vi "LJM_ListAllS.vi"(8 "error in":errorcluster, 10 "ConnectionType":string="LJM_ctUSB", 11 "DeviceType":string="LJM_dtT7") -> (0 "error out":errorcluster, 1 "aIPAddresses (IPv4Strings)":string[](array[string]), 2 "aIPAddresses":i32[](array[numeric]), 3 "aSerialNumbers":i32[](array[numeric]), 4 "aConnectionTypes":i32[](array[numeric]), 5 "NumFound":i32, 6 "aDeviceTypes":i32[](array[numeric]))   [LabVIEW 2020]
uses:
  LabJackM.framework
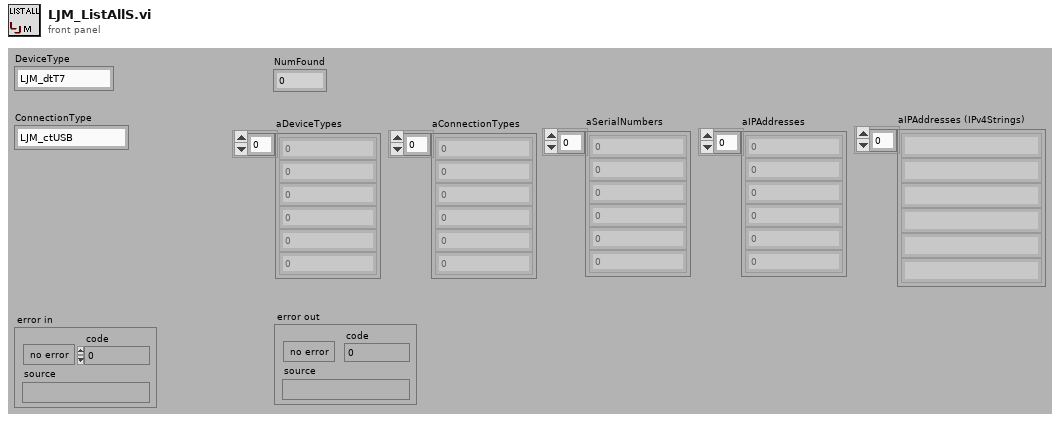
[diagram p1: front panel]
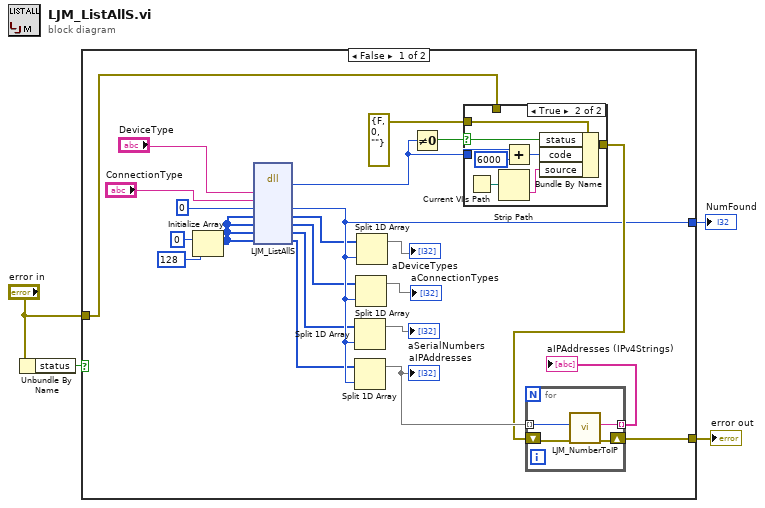
[diagram p0: block diagram]
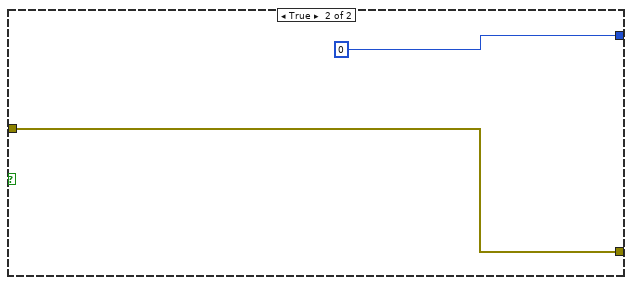
[diagram p3: hidden frame]
diagram:
  n1 = Unbundle By Name("error in") -> ("status"=w4:bool)
  n2 = case shown="False" w4 {
    tunnel: "error in" -> [w23 w41]
    tunnel: [w11 0 ("NumFound")] -> w2
    tunnel: [w13 w41] -> w1
    frame False {
      n3 = Initialize Array(0 ("element"), 128 ("dimension size")) -> (w12:i32[])
      n4 = dll-call lib="LabJackM.framework" fn="LJM_ListAllS"("DeviceType"="DeviceType", "ConnectionType"="ConnectionType", "NumFound"=0 ("Handle"), "aDeviceTypes"=w12, "aConnectionTypes"=w12, "aIPAddresses"=w12, "aSerialNumbers"=w12) -> ("return type"=w24:i32, "NumFound"=w11:i32, "aDeviceTypes"=w7:i32[], "aConnectionTypes"=w8:i32[], "aIPAddresses"=w9:i32[], "aSerialNumbers"=w10:i32[])  [unwired: 5 in, 2 out]
      n5 = Split 1D Array(array=w9, index=w11) -> (first subarray=→"aSerialNumbers":i32[])  [unwired: 1 out]
      n6 = Split 1D Array(array=w10, index=w11) -> (first subarray=w16:i32[])  [unwired: 1 out]
      "aIPAddresses" <- w16
      n7 = Split 1D Array(array=w8, index=w11) -> (first subarray=→"aConnectionTypes":i32[])  [unwired: 1 out]
      n8 = Split 1D Array(array=w7, index=w11) -> (first subarray=→"aDeviceTypes":i32[])  [unwired: 1 out]
      n9 = Not Equal To 0?(x=w24) -> (x != 0?=w25:bool)
      n10 = case shown="True" w25 {
        selector: w25 -> [_ w38]
        tunnel: [w31 w39] -> w14
        tunnel: errorcluster {"status"=FALSE, "code"=0, "source"=""} ("error IO") -> [_ w37]
        tunnel: w24 -> [_ w33]
        tunnel: w23 -> [w31 _]
        frame False {
        }
        frame True {
          n11 = Current VI's Path() -> (path=w35:path)
          n12 = Strip Path(path=w35) -> (name=w36:string)  [unwired: 1 out]
          n13 = Add(x=w33, y=6000) -> (x+y=w34:i32)
          n14 = Bundle By Name(cluster=w37, "status"=w38, "code"=w34, "source"=w36) -> (w39:errorcluster)
        }
      }
      n15 = for {
        tunnel: w16 -> [w30] mode=indexing
        tunnel: [w29] -> w15 mode=indexing
        shift-right: [w27] -> w13
        shift-left: w14 -> [w28]
        n16 = call "LJM_NumberToIP.vi"("error in"=w28, "Number"=w30) -> ("error out"=w27:errorcluster, "IPv4String"=w29:string)  [unwired: 8 in]
      }
      "aIPAddresses (IPv4Strings)" <- w15
    }
    frame True {
    }
  }
  "error out" <- w1
  "NumFound" <- w2
